vi "Processing Step.vi"(8 "error in (no error)":errorcluster, 11 "Authentication Handler in":refnum<class "Authentication Handler.lvclass">) -> (0 "error out":errorcluster, 2 "Step":T1[](array[typedef]), 3 "Authentication Handler out":refnum<class "Authentication Handler.lvclass">)   [LabVIEW 2020, in "HTTP Server.lvlib" / "Authentication Handler.lvclass"]
uses:
  Authentication Handler.lvclass
  Processing Step.ctl
  HTTP Server.lvlib
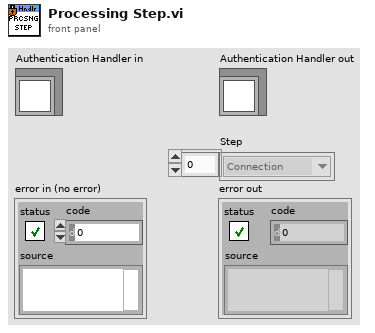
[diagram p1: front panel]
types:
  T1 = typedef "HTTP Server.lvlib/Processing Step.ctl" = enum16{"Connection", "Request", "Routing", "Controller Init", "Controller", "Response", "Complete", "Exception"}
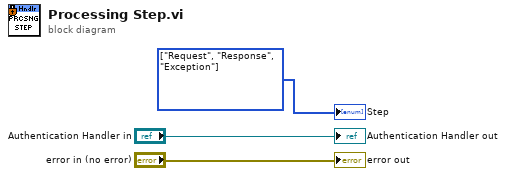
[diagram p0: block diagram]
diagram:
  w1 = T1[] [enum."Request", enum."Response", enum."Exception"] items=["Connection", "Request", "Routing", "Controller Init", "Controller", "Response", "Complete", "Exception"] ("Step")
  "error out" <- "error in (no error)"
  "Authentication Handler out" <- "Authentication Handler in"
  "Step" <- w1
